vi "lsl wait for consumers.vi"(8 "error in (no error)":errorcluster, 10 "timeout":dbl, 11 "outlet":T1) -> (0 "error out":errorcluster, 3 "wait for consumers":i32)   [LabVIEW 2018, in "liblsl-LabVIEW.lvlib"]
doc: "extern LIBLSL_C_API int32_t lsl_wait_for_consumers(lsl_outlet out, double timeout);"
uses:
  <userlib>/liblsl-LabVIEW/liblsl-LabVIEW.lvlib
  <userlib>/liblsl-LabVIEW/Custom Controls/lsl_outlet.ctl
  <userlib>/liblsl-LabVIEW/liblsl64.dll
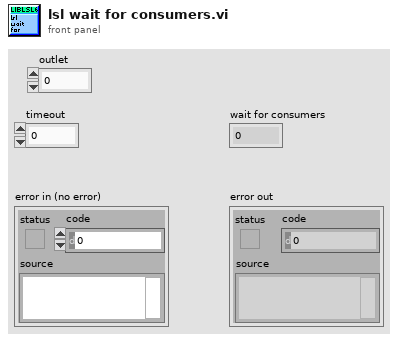
[diagram p1: front panel]
types:
  T1 = typedef "liblsl-LabVIEW.lvlib/lsl_outlet.ctl" = u64
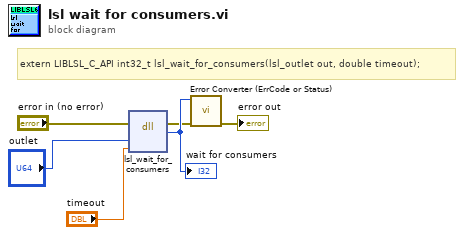
[diagram p0: block diagram]
diagram:
  # "extern LIBLSL_C_API int32_t lsl_wait_for_consumers(lsl_outlet out, double timeout);"
  n1 = dll-call lib="C:/Program Files/National Instruments/LabVIEW 2018/user.lib/liblsl-LabVIEW/liblsl64.*" fn="lsl_wait_for_consumers"(error in="error in (no error)", "out"="outlet", "timeout"="timeout") -> (error out=w3:errorcluster, "return type"=w6:i32)  [unwired: 4 in, 1 out]
  "wait for consumers" <- w6
  n2 = call <userlib>:"Error Converter (ErrCode or Status).vi"("error in (no error)"=w3, "error code"=w6) -> ("error out"=→"error out":errorcluster)  [unwired: 9 in]
